vi "Player Info.vi"(8 "Victory Speech":string="So you think you can dance?", 9 "Name":string="Line Dancer", 11 "Line Dancer in":refnum<class "Line Dancer.lvclass">) -> (3 "Line Dancer out":refnum<class "Line Dancer.lvclass">)   [LabVIEW 2015, in "Line Dancer.lvclass"]
uses:
  Line Dancer.lvclass
  Square/Square.lvclass
panel:
  # "Set default values for these two string controls"
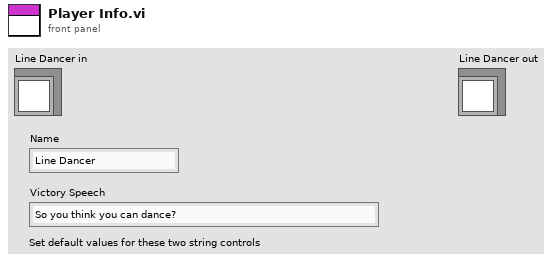
[diagram p1: front panel]
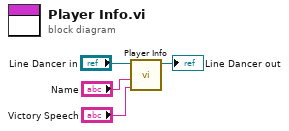
[diagram p0: block diagram]
diagram:
  n1 = call-parent "Player Info.vi"("Victory Speech"="Victory Speech", "Name"="Name", "Square in"="Line Dancer in") -> ("Square out"=→"Line Dancer out":refnum<class "Line Dancer.lvclass">)  [unwired: 8 in]
